vi "Create File Dependency.vi"(8 "error in (no error)":errorcluster, 9 "DLL Path":path, 10 "DLL Property Name":string, 11 "Item Ref in":T1 format="%.0x") -> (0 "error out":errorcluster, 3 "Item Ref out":T1 format="%.0x")   [LabVIEW 2015, in "Diagnostics Addon System Explorer.lvlib"]
uses:
  Diagnostics Addon System Explorer.lvlib
  <vilib>/NI Veristand/Custom Device API/Custom Device Item Ref.ctl
  <vilib>/NI Veristand/Custom Device API/Dependent File Optional Info.ctl
  <vilib>/NI Veristand/Custom Device API/Set Item Property (Dependent File).vi
  Shared/SubVIs/GUID Lookup.vi
  <vilib>/NI Veristand/Custom Device API/Custom Device API.lvlib
  Shared/Diagnostics Addon Shared.lvlib
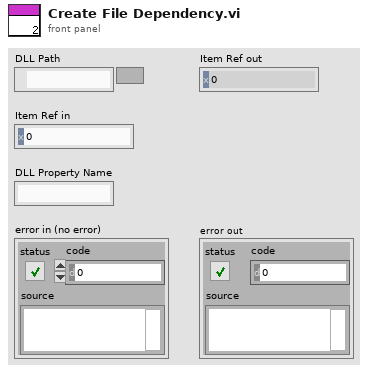
[diagram p1: front panel]
types:
  T1 = typedef "Custom Device API.lvlib/Custom Device Item Ref.ctl" = u64
  T2 = typedef "Custom Device API.lvlib/Dependent File Optional Info.ctl" = cluster{"Version":string, "RTDestination":path, "ForceDownload":bool, "SupportedTarget":string, "MD5":string}
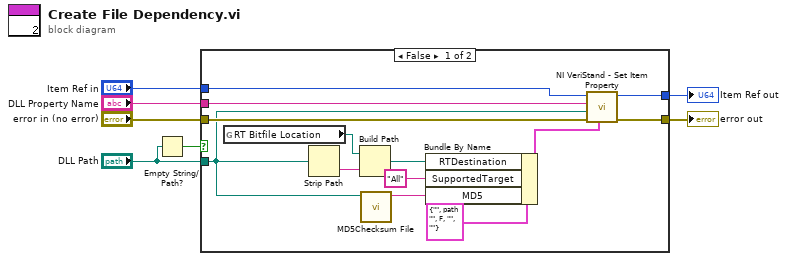
[diagram p0: block diagram]
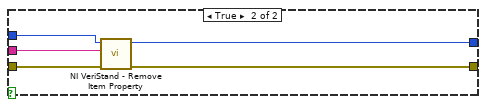
[diagram p2: hidden frame]
diagram:
  n1 = Empty String/Path?(string/path="DLL Path") -> (empty?=w6:bool)
  n2 = case shown="False" w6 {
    tunnel: "error in (no error)" -> [w20 w24]
    tunnel: [w19 w23] -> w3
    tunnel: [w18 w22] -> w4
    tunnel: "Item Ref in" -> [w17 w25]
    tunnel: "DLL Property Name" -> [w16 w21]
    tunnel: "DLL Path" -> [w9 _]
    frame False {
      n3 = global read "GUID Lookup.vi" "RT Bitfile Location"() -> (w15:path)
      n4 = Strip Path(path=w9) -> (name=w14:string)  [unwired: 1 out]
      n5 = Build Path(base path=w15, name or relative path=w14) -> (appended path=w12:path)
      n6 = call <vilib>:"MD5Checksum File.vi"("Path"=w9) -> ("MD5 message-digest"=w8:string)  [unwired: 9 in, 1 out]
      n7 = Bundle By Name(cluster=T2 {"Version"="", "RTDestination"=path "", "ForceDownload"=FALSE, "SupportedTarget"="", "MD5"=""} ("OptionalInfo"), "RTDestination"=w12, "SupportedTarget"="All", "MD5"=w8) -> (w11:T2)
      n8 = call-poly <vilib>:"NI VeriStand - Set Item Property.vi"("OptionalInfo"=w11, "error in (no error)"=w20, "Path"=w9, "Property Name"=w16, "Item Ref in"=w17) -> ("error out"=w19:errorcluster, "Item Ref out"=w18:T1)  [unwired: 4 in, 1 out]
    }
    frame True {
      n9 = call <vilib>:"NI VeriStand - Remove Item Property.vi"("error in (no error)"=w24, "Property Name"=w21, "Item Ref in"=w25) -> ("error out"=w23:errorcluster, "Item Ref out"=w22:T1)  [unwired: 6 in, 1 out]
    }
  }
  "Item Ref out" <- w4
  "error out" <- w3
